vi "UT_LV to TOML_001.vi"() -> ()   [LabVIEW 2017]
uses:
  <vilib>/addons/_JKI Toolkits/Caraya/classes/Assert/Assert True.vi
  <vilib>/addons/_JKI Toolkits/Caraya/classes/Assert/Assert Error.vi
  <vilib>/addons/_JKI Toolkits/Caraya/classes/Test/Test.lvclass
  <vilib>/addons/_JKI Toolkits/Caraya/classes/Assert/Assert.lvclass
  lib/TOML.lvlib
panel:
  out "error out":errorcluster
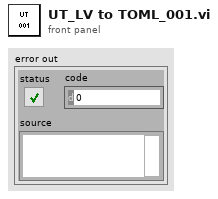
[diagram p1: front panel]
types:
  T1 = cluster{"error":cluster{"sttus":bool, "code":i32, "source":string}}
  T2 = typedef "TOML.lvlib/TOML Value.ctl" = cluster{"type":enum16{"Table", "Array", "String", "Integer", "Float", "Boolean", "Offset Date-Time", "Local Date-Time", "Local Date", "Local Time"}, "value":variant}
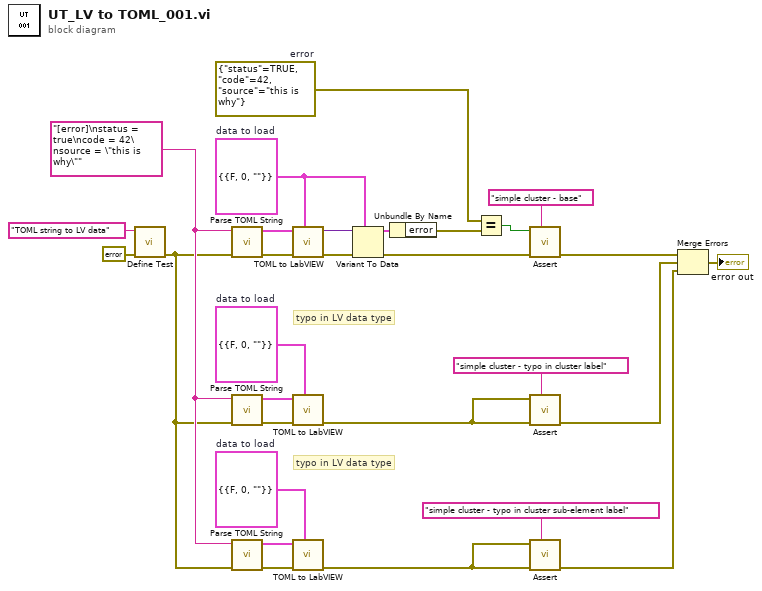
[diagram p0: block diagram]
diagram:
  w4 = T1 {"error"={"sttus"=FALSE, "code"=0, "source"=""}}  # data to load
  w14 = cluster{"errr":errorcluster} {"errr"={"status"=FALSE, "code"=0, "source"=""}}  # data to load
  w16 = cluster{"error":errorcluster} {"error"={"status"=FALSE, "code"=0, "source"=""}}  # data to load
  w19 = errorcluster {"status"=TRUE, "code"=42, "source"="this is why"}  # error
  w3 = "[error]\nstatus = true\ncode = 42\nsource = \"this is why\"" ("String")
  # "typo in LV data type"
  # "typo in LV data type"
  n1 = call <vilib>:"Define Test.vi"("error in (no error)"=errorcluster {"status"=FALSE, "code"=0, "source"=""}, "Label (VI Title)"="TOML string to LV data") -> ("error out"=w2:errorcluster)  [unwired: 9 in]
  n2 = call "Parse TOML String.vi"("error in (no error)"=w2, "String"=w3) -> ("error out"=w25:errorcluster, "Value"=w24:T2)  [unwired: 8 in]
  n3 = call "Parse TOML String.vi"("error in (no error)"=w2, "String"=w3) -> ("error out"=w12:errorcluster, "Value"=w13:T2)  [unwired: 8 in]
  n4 = call "Parse TOML String.vi"("error in (no error)"=w2, "String"=w3) -> ("error out"=w6:errorcluster, "Value"=w5:T2)  [unwired: 8 in]
  n5 = call "TOML to LabVIEW.vi"("Default Value"=w16, "error in (no error)"=w25, "TOML Value"=w24) -> ("error out"=w23:errorcluster, "LV Value"=w21:variant)  [unwired: 7 in]
  n6 = call "TOML to LabVIEW.vi"("Default Value"=w14, "error in (no error)"=w12, "TOML Value"=w13) -> ("error out"=w9:errorcluster)  [unwired: 7 in, 1 out]
  n7 = call "TOML to LabVIEW.vi"("Default Value"=w4, "error in (no error)"=w6, "TOML Value"=w5) -> ("error out"=w8:errorcluster)  [unwired: 7 in, 1 out]
  n8 = Variant To Data(error in=w23, type=w16, Variant=w21) -> (data=w20:cluster{"error":errorcluster}, error out=w22:errorcluster)
  n9 = Unbundle By Name(w20) -> ("error"=w15:errorcluster)
  n10 = Equal?(x=w19, y=w15) -> (x = y?=w18:bool)
  n11 = call-poly <vilib>:"Assert.vi"("Label"="simple cluster - base" ("Label (VI Title)"), "error in (no error)"=w22, "True?"=w18) -> ("error out"=w28:errorcluster)  [unwired: 8 in]
  n12 = call-poly <vilib>:"Assert.vi"("Label"="simple cluster - typo in cluster label" ("Label (VI Title)"), "error in (no error)"=w9, "Error?"=w9) -> ("error out"=w10:errorcluster)  [unwired: 8 in]
  n13 = call-poly <vilib>:"Assert.vi"("Label"="simple cluster - typo in cluster sub-element label" ("Label (VI Title)"), "error in (no error)"=w8, "Error?"=w8) -> ("error out"=w1:errorcluster)  [unwired: 8 in]
  n14 = Merge Errors(w28, w10, w1) -> (→"error out":errorcluster)
